vi "SQLSetEnvAttr.vi"(4 "error in (no error)":errorcluster, 5 "AttributeValue":u32, 6 "AttributePosition":i32, 7 "InputHandle":i32) -> (0 "error out":errorcluster, 3 "OutputHandle":i32)   [LabVIEW 2011]
doc: "Configure l'environnement en fonction des paramètres d'entrée"
uses:
  Odbc32.dll
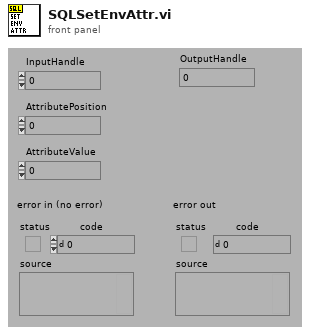
[diagram p1: front panel]
types:
  T1 = enum16{"NOPE", "SQL_HANDLE_ENV", "SQL_HANDLE_DBC", "SQL_HANDLE_STMT", "SQL_HANDLE_DESC"}
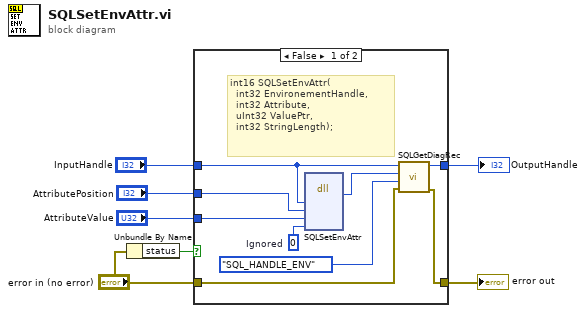
[diagram p0: block diagram]
diagram:
  n1 = Unbundle By Name("error in (no error)") -> ("status"=w1:bool)
  n2 = case shown="False" w1 {
    tunnel: "AttributePosition" -> [w16 _]
    tunnel: "AttributeValue" -> [w15 _]
    tunnel: "error in (no error)" -> [w13 w17]
    tunnel: [w11 w18] -> w4
    tunnel: "InputHandle" -> [w10 w18]
    tunnel: [w9 w17] -> w2
    frame False {
      w14 = 0  # Ignored
      # "int16 SQLSetEnvAttr(\n  int32 EnvironementHandle, \n  int32 Attribute, \n  uInt32 ValuePtr, \n  int32 StringLength);"
      n3 = dll-call lib="Odbc32.dll" fn="SQLSetEnvAttr"("EnvironementHandle"=w10, "Attribute"=w16, "ValuePtr"=w15, "StringLength"=w14) -> (w12:i16)  [unwired: 7 in, 2 out]
      n4 = call "SQLGetDiagRec.vi"("error in (no error)"=w13, "HandleType"=T1."SQL_HANDLE_ENV", "Status (SQL_SUCCESS=0)"=w12, "Input Handle"=w10) -> ("error out"=w9:errorcluster, "Output Handle"=w11:i32)  [unwired: 2 out]
    }
    frame True {
    }
  }
  "OutputHandle" <- w4
  "error out" <- w2
